vi "Read Ramp Parameters.vi"(8 "error in (no error)":errorcluster, 11 "signal configuration":refnum<class "SV Signal.lvclass">) -> (0 "error out":errorcluster, 2 "ramp parameters":T1 {"durations [s]"."ramp-down" format="%.2p"; "durations [s]"."transition" format="%.2p"; "durations [s]"."ramp-up" format="%.2p"}, 3 "signal configuration":refnum<class "SV Signal.lvclass">)   [LabVIEW 2017, in "SV Signal.lvclass"]
uses:
  <vilib>/addons/_NISVFA/_Generation/Signal Generation/SV Signal/SV Signal.lvclass
  <vilib>/addons/_NISVFA/_Generation/Signal Generation/SV Signal/SV Signal.lvclass/SV Signal.ctl
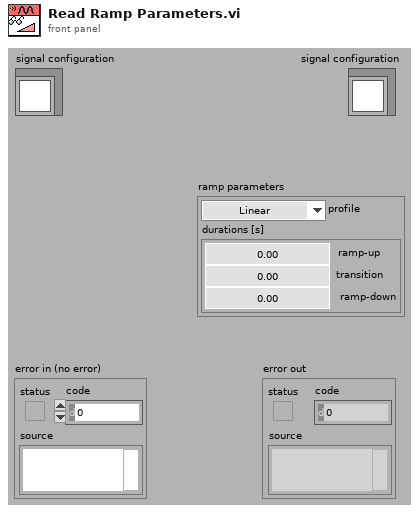
[diagram p1: front panel]
types:
  T1 = cluster{"profile":enum16{"Linear", "Half cosine"}, "durations [s]":cluster{"ramp-up":dbl, "transition":dbl, "ramp-down":dbl}}
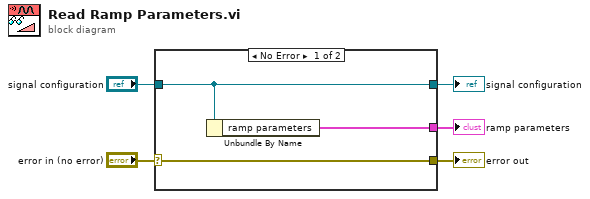
[diagram p0: block diagram]
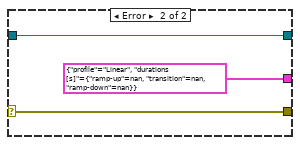
[diagram p2: hidden frame]
diagram:
  n1 = case shown="No Error" "error in (no error)" {
    selector: "error in (no error)" -> [w8 w10]
    tunnel: [w8 w10] -> w4
    tunnel: [w7 w11] -> w2
    tunnel: "signal configuration" -> [w7 w11]
    tunnel: [w6 T1 {"profile"=enum."Linear", "durations [s]"={"ramp-up"=nan, "transition"=nan, "ramp-down"=nan}} ("ramp parameters")] -> w1
    frame No Error {
      n2 = Unbundle By Name(w7) -> ("ramp parameters"=w6:T1)
    }
    frame Error {
    }
  }
  "error out" <- w4
  "signal configuration" <- w2
  "ramp parameters" <- w1
